vi "GeneralControlFIFO.vi"   [LabVIEW 2016]
uses:
  <vilib>/rvi/DataTransferAndStorage/Container/XNode/niFpgaContainer.xnode
  Common_FPGA_FIFO/FPGAFIFO.lvlib
  <vilib>/rvi/interface/RandomDataEmulation/nirviRandomDataFpgaReadWriteTemplate.vi
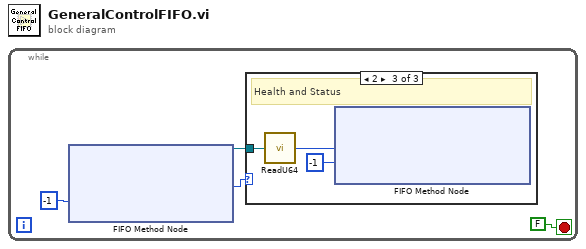
[diagram p0: block diagram]
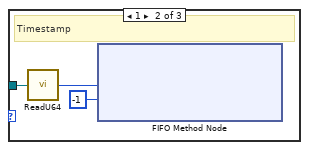
[diagram p3: hidden frame]
diagram:
  n1 = while {
    stop <- FALSE stop-if-true
    n2 = xnode ("FIFO Method Node")("Timeout"=-1) -> ("Element"=w2:u8, "FIFO Out"=w1:refnum<k21>)  [unwired: 1 in, 1 out]
    n3 = case shown="2" w2 {
      tunnel: w1 -> [_ w7 w10]
      frame 0, Default {
      }
      frame 1 {
        # "Timestamp"
        n4 = call "ReadU64.vi"("FIFO"=w7) -> ("U64"=w6:u64)
        n5 = xnode ("FIFO Method Node")("Element"=w6, "Timeout"=-1) -> ()  [unwired: 1 in, 2 out]
      }
      frame 2 {
        # "Health and Status"
        n6 = call "ReadU64.vi"("FIFO"=w10) -> ("U64"=w9:u64)
        n7 = xnode ("FIFO Method Node")("Element"=w9, "Timeout"=-1) -> ()  [unwired: 1 in, 2 out]
      }
    }
  }
